vi "Configure.vi"(8 "error in (no error)":errorcluster, 10 "Configuration":T1={"mode"=enum."AC_Current", "Range"=0.0, "Resolution"=0.0}, 11 "VISA resource name":refnum<visa-resource-name>) -> (0 "error out":errorcluster, 3 "VISA resource name out":refnum<visa-resource-name>)   [LabVIEW 2023, in "Keysight-34450A.lvlib"]
doc: "<b>Author:</b> Wolfgang\n<b>Description:</b> Configure measurement type and range."
uses:
  Keysight-34450A.lvlib
  TypeDef/configuration.ctl
  TypeDef/mode.ctl
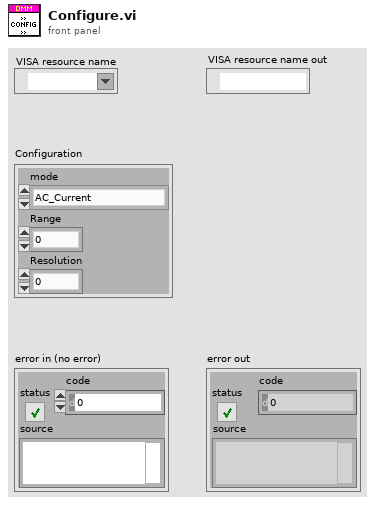
[diagram p1: front panel]
types:
  T1 = typedef "Keysight-34450A.lvlib/configuration.ctl" = cluster{"mode":T2, "Range":dbl, "Resolution":dbl}
  T2 = typedef "Keysight-34450A.lvlib/mode.ctl" = enum16{"DC_Voltage", "AC_Voltage", "DC_Current", "AC_Current", "Resistance"}
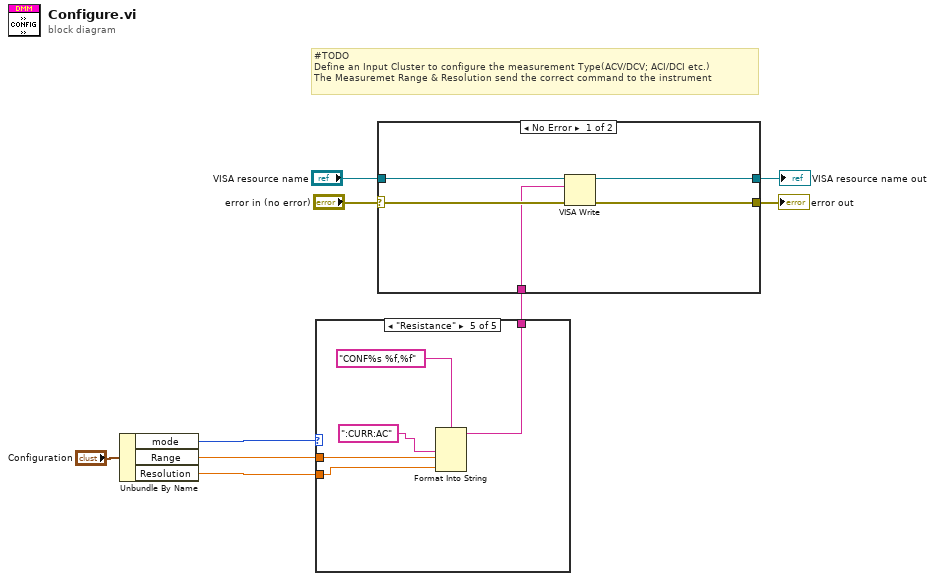
[diagram p0: block diagram]
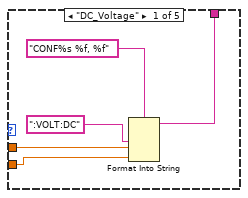
[diagram p2: hidden frame]
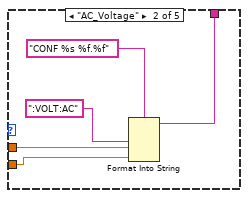
[diagram p3: hidden frame]
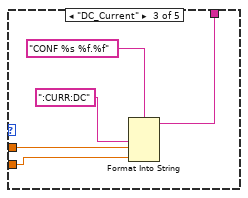
[diagram p4: hidden frame]
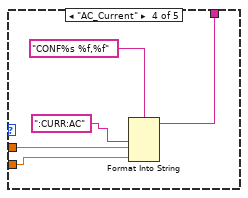
[diagram p5: hidden frame]
diagram:
  # "#TODO\nDefine an Input Cluster to configure the measurement Type(ACV/DCV; ACI/DCI etc.)\nThe Measuremet Range & Resolution send the correct command to the instrument"
  n1 = Unbundle By Name("Configuration") -> ("mode"=w3:T2, "Range"=w2:dbl, "Resolution"=w1:dbl)
  n2 = case shown="\"Resistance\"" w3 {
    tunnel: [w13 w18 w23 w28 w33] -> w5
    tunnel: w2 -> [w12 w17 w22 w27 w32]
    tunnel: w1 -> [w11 w16 w21 w26 w31]
    frame "DC_Voltage" {
      n3 = Format Into String(format string="CONF%s %f, %f", ":VOLT:DC", w12, w11) -> (resulting string=w13:string)  [unwired: 2 in, 1 out]
    }
    frame "AC_Voltage" {
      n4 = Format Into String(format string="CONF %s %f.%f", ":VOLT:AC" ("initial string"), w17, w16) -> (resulting string=w18:string)  [unwired: 2 in, 1 out]
    }
    frame "DC_Current" {
      n5 = Format Into String(format string="CONF %s %f.%f", ":CURR:DC" ("initial string"), w22, w21) -> (resulting string=w23:string)  [unwired: 2 in, 1 out]
    }
    frame "AC_Current" {
      n6 = Format Into String(format string="CONF%s %f,%f", ":CURR:AC" ("initial string"), w27, w26) -> (resulting string=w28:string)  [unwired: 2 in, 1 out]
    }
    frame "Resistance" {
      n7 = Format Into String(format string="CONF%s %f,%f", ":CURR:AC" ("initial string"), w32, w31) -> (resulting string=w33:string)  [unwired: 2 in, 1 out]
    }
  }
  n8 = case shown="No Error" "error in (no error)" {
    selector: "error in (no error)" -> [w36 w41]
    tunnel: [w38 w40] -> w9
    tunnel: [w39 w41] -> w7
    tunnel: "VISA resource name" -> [w37 w40]
    tunnel: w5 -> [w35 _]
    frame No Error {
      n9 = VISA Write(VISA resource name=w37, write buffer=w35, error in (no error)=w36) -> (VISA resource name out=w38:refnum<visa-resource-name>, error out=w39:errorcluster)  [unwired: 1 out]
    }
    frame Error {
    }
  }
  "VISA resource name out" <- w9
  "error out" <- w7
